vi "AG33XXX.reset.vi"(0 "i ref in":refnum<vi>, 3 "ms timeout (10000)":i32=10000, 5 "error in (no error)":errorcluster) -> (14 "i ref out":refnum<vi>, 17 "timed out":bool, 19 "error out":errorcluster)   [LabVIEW 2014, in "AG33XXX.lvlib"]
doc: "Resets the device and enables the output."
uses:
  AG33XXX.lvlib
  CSCore/CSApplicationBaseClasses/AFGBase/AFGBase.waveformType.ctl
  CSlibraries/UtilityLib/UtilityLib.valueStatus.ctl
  CSCore/CSApplicationBaseClasses/DeviceBase/DeviceBase.lvlib
  CSCore/CSApplicationBaseClasses/AFGBase/AFGBase.lvlib
  CSinstr.lib/Agilent 33xxx Series/Agilent 33XXX Series.lvlib
  CSlibraries/UtilityLib/UtilityLib.lvlib
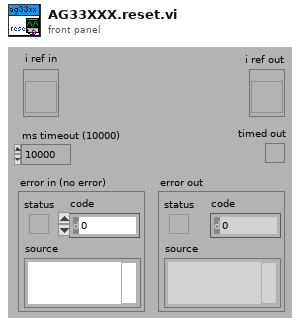
[diagram p1: front panel]
types:
  T1 = typedef "UtilityLib.lvlib/UtilityLib.valueStatus.ctl" = enum16{"no info available", "stand by/off", "on", "warning", "alarm/malfunction", "not implemented", "user action required", "important information", "system default", "control default", "indicator default", "button default"}
  T2 = typedef "AFGBase.lvlib/AFGBase.waveformType.ctl" = enum16{"sine", "square", "ramp", "pulse", "noise", "DC", "arbitrary", "triangle", "ramp_up", "ramp_down", "amplitude modulation"}
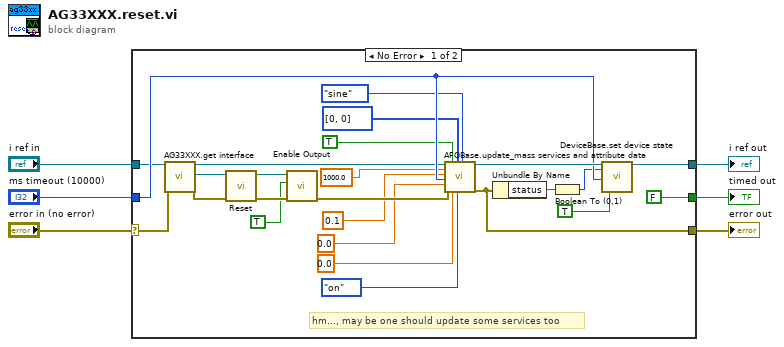
[diagram p0: block diagram]
diagram:
  n1 = case shown="No Error" "error in (no error)" {
    selector: "error in (no error)" -> [w22 w32]
    tunnel: [FALSE _] -> w6
    tunnel: [w29 w33] -> w5
    tunnel: "ms timeout (10000)" -> [w26 _]
    tunnel: "i ref in" -> [w23 w33]
    tunnel: [w27 w32] -> w1
    frame No Error {
      # "hm..., may be one should update some services too"
      n2 = call "AG33XXX.get interface.vi"("i ref in"=w23, "error in (no error)"=w22) -> ("i ref out"=w19:refnum<vi>, "interface"=w21:refnum<visa-resource-name>, "error out"=w20:errorcluster)  [unwired: 15 in]
      n3 = call "Reset.vi"("error in (no error)"=w20, "VISA resource name"=w21) -> ("error out"=w17:errorcluster, "VISA resource name out"=w18:refnum<visa-resource-name>)  [unwired: 8 in]
      n4 = call "Enable Output.vi"("error in (no error)"=w17, "Enable Output (T: Enable)"=TRUE, "VISA resource name"=w18) -> ("error out"=w15:errorcluster)  [unwired: 7 in, 1 out]
      n5 = call "AFGBase.update_mass services and attribute data.vi"("i ref in"=w19, "frequency"=1000.0, "amplitude"=0.1, "ms timeout (10000)"=w26, "phase"=0.0, "error in (no error)"=w15, "enableOutput"=TRUE, "DCOffset"=0.0, "trigger"=i16[] [0, 0], "valueStatus"=UtilityLib.valueStatus."on", "waveformType"=AFGBase.waveformType."sine") -> ("i ref out"=w28:refnum<vi>, "error out"=w27:errorcluster)  [unwired: 6 in, 1 out]
      n6 = Unbundle By Name(w27) -> ("status"=w30:bool)
      n7 = Boolean To (0,1)(Boolean=w30) -> (0, 1=w25:i16)
      n8 = call "DeviceBase.set device state.vi"("i ref in"=w28, "deviceState"=w25, "ms timeout (10000)"=w26, "mayResetError (FALSE)"=TRUE) -> ("i ref out"=w29:refnum<vi>)  [unwired: 13 in, 2 out]
    }
    frame Error {
    }
  }
  "error out" <- w1
  "i ref out" <- w5
  "timed out" <- w6
